vi "Depth2ColorImage.vi"(11 "Depth":u16[][](array[numeric])) -> (3 "HSV Image":picture)   [LabVIEW 2015]
uses:
  <vilib>/picture/picture.llb/Draw True-Color Pixmap.vi
panel:
  out "Array 2":u16[][](array[ring])
  out "Array":dbl[][](array[numeric])
  out "p":dbl
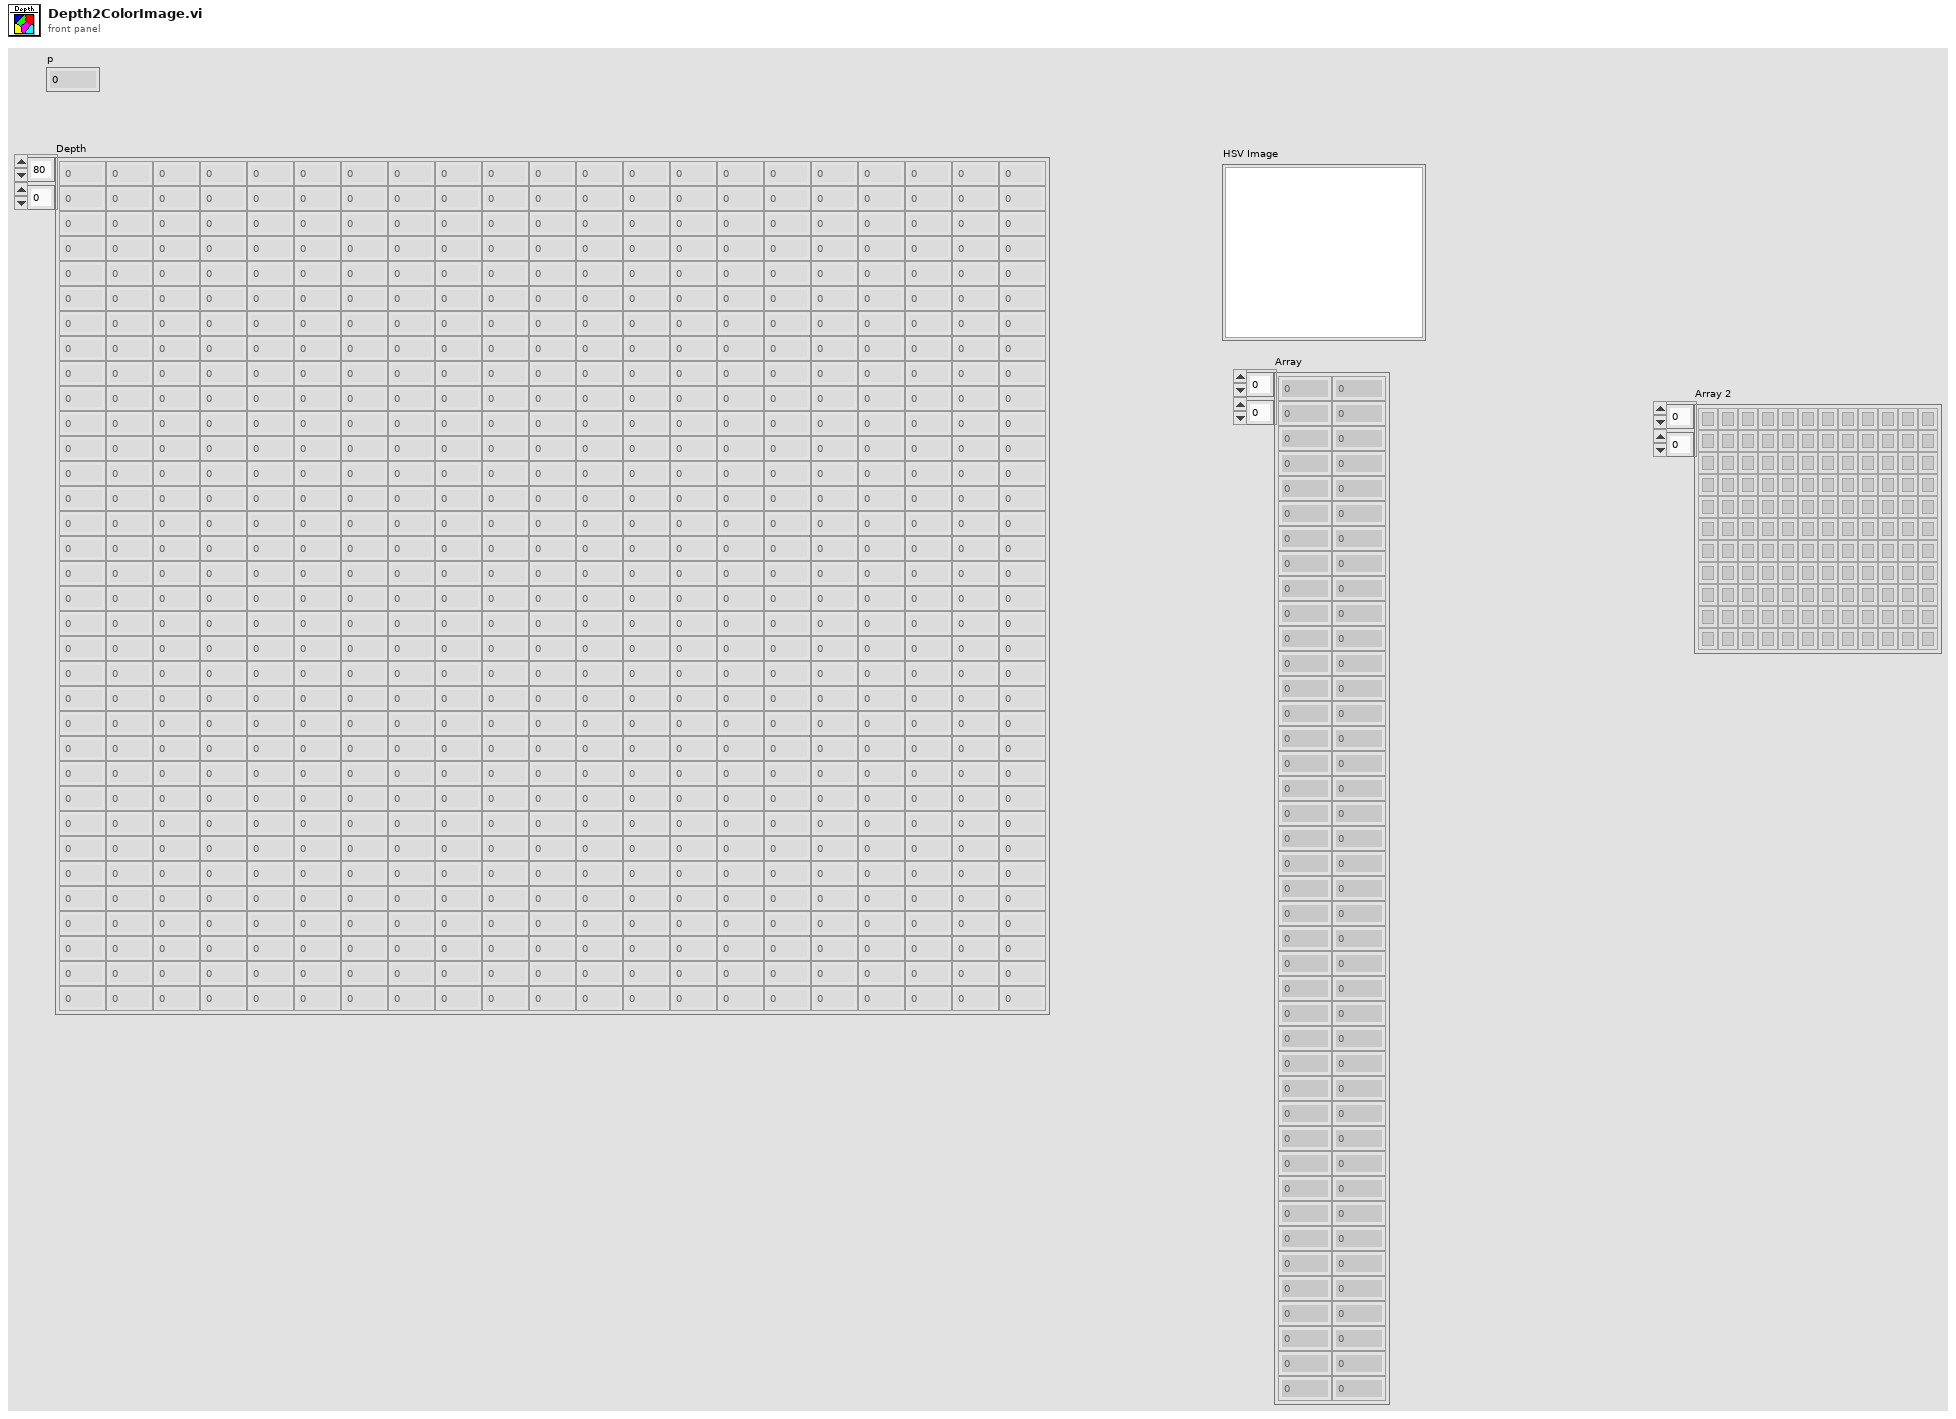
[diagram p1: front panel]
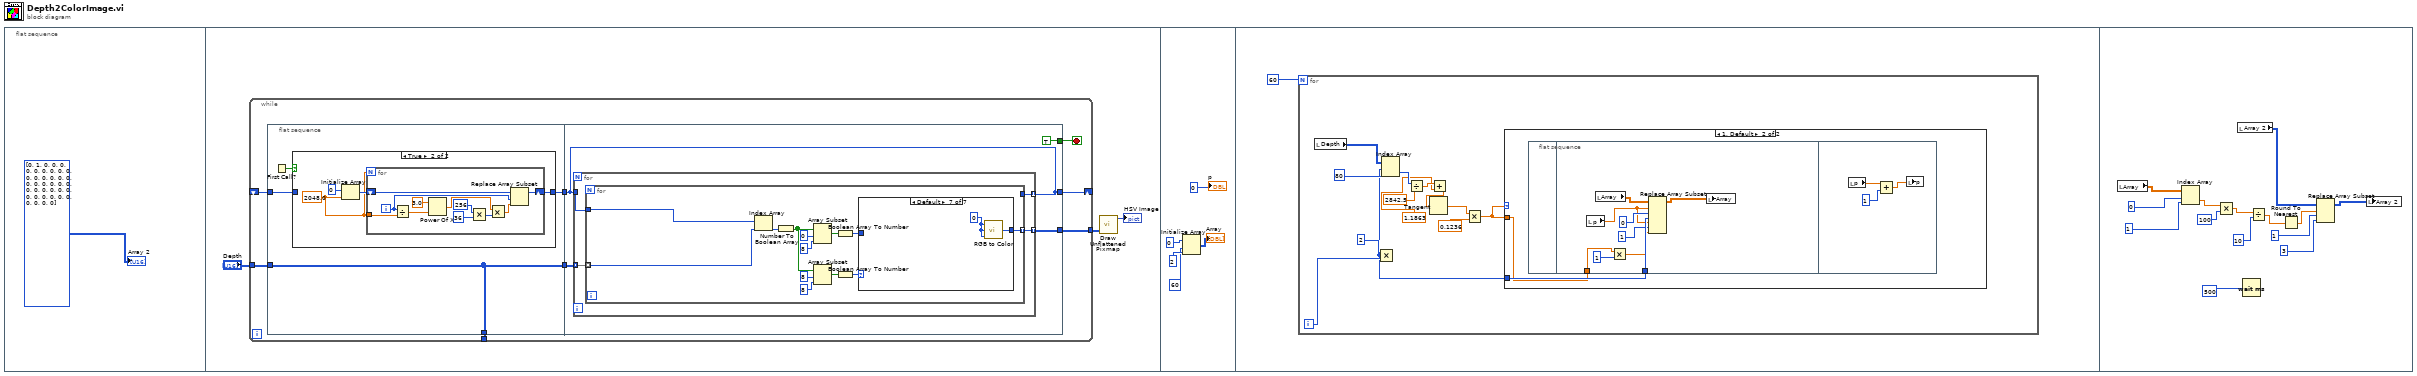
[diagram p0: block diagram]
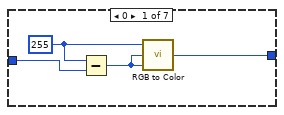
[diagram p3: hidden frame]
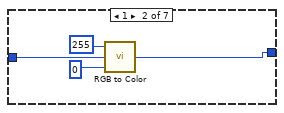
[diagram p4: hidden frame]
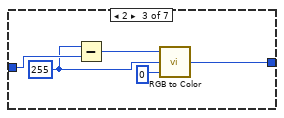
[diagram p5: hidden frame]
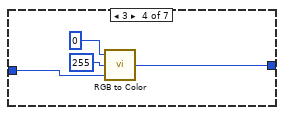
[diagram p6: hidden frame]
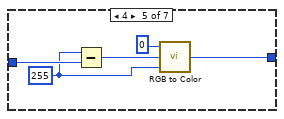
[diagram p7: hidden frame]
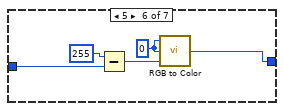
[diagram p8: hidden frame]
diagram:
  n1 = flat-sequence {
    frame #0 {
      "Array 2" <- i32[][] [[0, 1, 0], [0, 0, 0], [0, 0, 0], [0, 0, 0], [0, 0, 0], [0, 0, 0], [0, 0, 0], [0, 0, 0], [0, 0, 0], [0, 0, 0], [0, 0, 0], [0, 0, 0], [0, 0, 0]]
    }
    frame #1 {
      n2 = while {
        shift-right: [w11] -> _
        shift-left: _ -> [w10]
        tunnel: "Depth" -> [w8]
        tunnel: [w6] -> w3
        tunnel: [w5] -> _
        stop <- w7 stop-if-true
        n3 = flat-sequence {
          tunnel: [w15] -> w12
          tunnel: w10 -> [w14]
          tunnel: [w13] -> w9
          tunnel: w8 -> [w13]
          tunnel: [w13] -> w5
          tunnel: w12 -> [w33]
          tunnel: [w33] -> w11
          tunnel: w9 -> [w36]
          tunnel: [TRUE] -> w7
          tunnel: [w34] -> w6
          frame #0 {
            n4 = First Call?() -> (First Call?: T/F=w16:bool)
            n5 = case shown="True" w16 {
              tunnel: [w17 w18] -> w15
              tunnel: w14 -> [w17 _]
              frame False {
              }
              frame True {
                w19 = 2048.0
                n6 = Initialize Array(u16 0 ("element"), w19) -> (w20:u16[])
                n7 = for {
                  N: w19 -> [_]
                  shift-right: [w23] -> w18
                  shift-left: w20 -> [w32]
                  tunnel: w19 -> [w30]
                  i -> [w31]
                  n8 = Divide(x=w31, y=w30) -> (x/y=w29:dbl)
                  n9 = Power Of X(1:w29, 2:3.0 ("y")) -> (0:w27:dbl)
                  n10 = Multiply(x=256, y=36) -> (x*y=w24:i32)
                  n11 = Multiply(x=w27, y=w24) -> (x*y=w22:dbl)
                  n12 = Replace Array Subset(array=w32, new element=w22, index=w31) -> (w23:u16[])
                }
              }
            }
          }
          frame #1 {
            n13 = for {
              tunnel: w36 -> [w40] mode=indexing
              tunnel: w33 -> [w39]
              tunnel: [w38] -> w34 mode=indexing
              tunnel: w33 -> [w37] mode=indexing
              n14 = for {
                tunnel: w40 -> [w42] mode=indexing
                tunnel: w39 -> [w53]
                tunnel: [w43] -> w38 mode=indexing
                tunnel: w37 -> [_]
                n15 = Index Array(array=w53, index=w42) -> (element=w41:u16)
                n16 = Number To Boolean Array(number=w41) -> (Boolean array=w50:bool[])
                n17 = Array Subset(array=w50, index=0, length=8) -> (w47:bool[])
                n18 = Array Subset(array=w50, index=8, length=8) -> (w46:bool[])
                n19 = Boolean Array To Number(Boolean array=w47) -> (number=w44:u32)
                n20 = Boolean Array To Number(Boolean array=w46) -> (number=w45:u32)
                n21 = case shown="Default" w45 {
                  tunnel: w44 -> [w56 w59 w66 w67 w73 w79 _]
                  tunnel: [w54 w60 w65 w70 w75 w80 w82] -> w43
                  frame 0 {
                    w57 = 255
                    n22 = Subtract(x=w57, y=w56) -> (x-y=w55:u32)
                    n23 = call <vilib>:"RGB to Color.vi"("B"=w55, "G"=w55, "R"=w57) -> ("Color"=w54:u32)
                  }
                  frame 1 {
                    n24 = call <vilib>:"RGB to Color.vi"("B"=0, "G"=w59, "R"=255) -> ("Color"=w60:u32)
                  }
                  frame 2 {
                    w63 = 255
                    n25 = Subtract(x=w63, y=w66) -> (x-y=w64:u32)
                    n26 = call <vilib>:"RGB to Color.vi"("B"=0, "G"=w63, "R"=w64) -> ("Color"=w65:u32)
                  }
                  frame 3 {
                    n27 = call <vilib>:"RGB to Color.vi"("B"=w67, "G"=255, "R"=0) -> ("Color"=w70:u32)
                  }
                  frame 4 {
                    w71 = 255
                    n28 = Subtract(x=w71, y=w73) -> (x-y=w72:u32)
                    n29 = call <vilib>:"RGB to Color.vi"("B"=w71, "G"=w72, "R"=0) -> ("Color"=w75:u32)
                  }
                  frame 5 {
                    w77 = 0
                    n30 = Subtract(x=255, y=w79) -> (x-y=w76:u32)
                    n31 = call <vilib>:"RGB to Color.vi"("B"=w76, "G"=w77, "R"=w77) -> ("Color"=w80:u32)
                  }
                  frame Default {
                    w81 = 0
                    n32 = call <vilib>:"RGB to Color.vi"("B"=w81, "G"=w81, "R"=w81) -> ("Color"=w82:u32)
                  }
                }
              }
            }
          }
        }
      }
      n33 = call-poly <vilib>:"Draw Unflattened Pixmap.vi"("data (RGB format)"=w3) -> ("new picture"=→"HSV Image":picture)  [unwired: 8 in]
    }
    frame #2 {
      n34 = Initialize Array(0, 60, 2) -> (→"Array":i32[][])
      "p" <- 0
    }
    frame #3 {
      n35 = for {
        N: 60 -> [_]
        i -> [w100]
        n36 = local read "Depth"() -> (w97:u16[][])
        n37 = Multiply(x=2, y=w100) -> (x*y=w98:i32)
        n38 = Index Array(array=w97, index (row)=w98, index (col)=80) -> (element=w93:u16)
        n39 = Divide(x=w93, y=2842.5) -> (x/y=w91:dbl)
        n40 = Add(x=w91, y=1.1863) -> (x+y=w90:dbl)
        n41 = Tangent(1:w90) -> (0:w94:dbl)
        n42 = Multiply(x=w94, y=0.1236) -> (x*y=w95:dbl)
        n43 = case shown="1, Default" w95 {
          tunnel: w98 -> [_ w103]
          tunnel: w95 -> [_ w102]
          frame 2047 {
          }
          frame 1, Default {
            n44 = flat-sequence {
              tunnel: w103 -> [w109]
              tunnel: w102 -> [w106]
              frame #0 {
              }
              frame #1 {
                n45 = local read "p"() -> (w108:dbl)
                n46 = local read "Array"() -> (w112:dbl[][])
                n47 = Multiply(x=w106, y=1) -> (x*y=w105:dbl)
                n48 = Replace Array Subset(array=w112, new element #1=w109, index (row) #1=w108, index (col) #1=0, new element #2=w105, index (row) #2=w108, index (col) #2=1) -> (w111:dbl[][])
                n49 = local write "Array"(w111) -> ()
              }
              frame #2 {
                n50 = local read "p"() -> (w113:dbl)
                n51 = Add(x=w113, y=1) -> (x+y=w114:dbl)
                n52 = local write "p"(w114) -> ()
              }
            }
          }
        }
      }
    }
    frame #4 {
      n53 = local read "Array"() -> (w129:dbl[][])
      n54 = Index Array(array=w129, index (row)=0, index (col)=1) -> (element=w126:dbl)
      n55 = Multiply(x=w126, y=100) -> (x*y=w124:dbl)
      n56 = local read "Array 2"() -> (w120:u16[][])
      n57 = Wait (ms)(milliseconds to wait=500) -> ()  [unwired: 1 out]
      n58 = Divide(x=w124, y=10) -> (x/y=w122:dbl)
      n59 = Round To Nearest(number=w122) -> (nearest integer value=w118:dbl)
      n60 = Replace Array Subset(array=w120, new element=3, index (row)=w118, index (col)=1) -> (w121:u16[][])
      n61 = local write "Array 2"(w121) -> ()
    }
  }
